vi "pulse_generator_multiheater_refnum_enable_modifier.vi"(1 "Disabled":T1(ring), 2 "DAQmxName Refnums":T2) -> ()   [LabVIEW 2015]
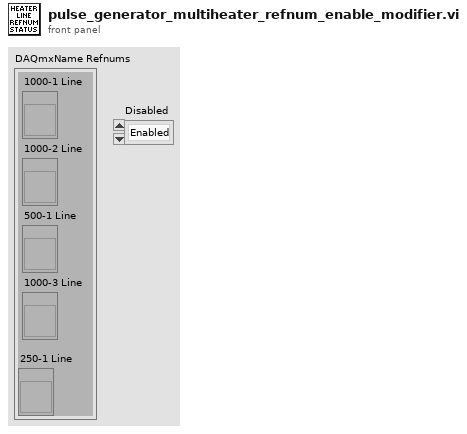
[diagram p1: front panel]
types:
  T1 = enum8{"Enabled", "Disabled", "Disabled and Grayed Out"}
  T2 = cluster{"1000-1 Line":refnum<vi>, "1000-2 Line":refnum<vi>, "1000-3 Line":refnum<vi>, "500-1 Line":refnum<vi>, "250-1 Line":refnum<vi>}
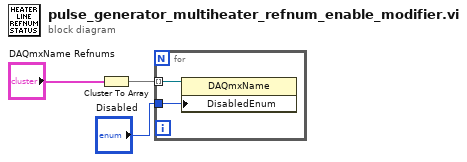
[diagram p0: block diagram]
diagram:
  n1 = Cluster To Array(cluster="DAQmxName Refnums") -> (array=w2:refnum<vi>[])
  n2 = for {
    tunnel: w2 -> [w5] mode=indexing
    tunnel: "Disabled" -> [w4]
    n3 = property class="DAQmxName"(reference=w5, "DisabledEnum"=w4) -> ()  [unwired: 1 in, 2 out]
  }
